vi "2ndStrikerNormal.vi"(5 "Stop":bool, 6 "atacando ao contrário?":bool=TRUE, 7 "AI Parameters":T1={"GotoKick"={"Dist do cone a frente"=150.0, "attacker farback"=1500.0, "Perto"=300.0, "min dist to kick"=150.0, "kick eps"=0.0, "Time to transition"=0.05}, "Attacker"={"CC chute"=0.09, "CC passe"=0.045, "Kick Force"=100.0, "ball-robot Kick"=200.0, "ball-robot Pass"=0.3, "drible\nAttk"=FALSE}, "Defender"={"D max"=1700.0, "Vel p/ robô av"=1000.0, "Kick Force"=100.0, "D atk-def"=0.0, "D farback"=0.0, "drible\ndef"=FALSE, "drible\ngoalie"=FALSE}, "Timeout"={"Field/v in x"=6.0, "Dist Robots"=300, "Dist up in y"=300}, "Pose Striker"={"dist"=200.0, "Numeric"=-4.0, "dist 2"=200.0, "drible\nstriker"=FALSE}, "Dist Stop"=300.0, "D ball out"=200, "D central gap "=150.0, "T pass"=0.0, "Force ++"=0.0, "range kick"=0.0, "Chute alto"=TRUE, "Marcador novo"=TRUE, "drible"=FALSE, "D drible"=300.0} {"D drible" format="%#_13g"; "D central gap" format="%#_13g"; "Dist Stop" format="%#_13g"; "Pose Striker"."Numeric" format="%#_13g"; "Defender"."Kick Force" format="%#_13g"; "Defender"."Vel p/ robô av" format="%#_13g"; "Attacker"."ball-robot Kick" format="%#_13g"; "Attacker"."Kick Force" format="%#_13g"; "Attacker"."CC passe" format="%#_13g"; "Attacker"."CC chute" format="%#_13g"; "GotoKick"."kick eps" format="%#_13g"; "GotoKick"."min dist to kick" format="%#_13g"; "GotoKick"."Perto" format="%#_13g"; "GotoKick"."attacker farback" format="%#_13g"; "GotoKick"."Dist do cone a frente" format="%#_13g"}, 8 "IA Input":T9={"our_robots"=[], "enemy_robots"=[], "balls"=[], "geometry"={"line_width"=0, "field_length"=0, "field_width"=0, "boundary_width"=0, "referee_width"=0, "goal_width"=0, "goal_depth"=0, "goal_wall_width"=0, "center_circle_radius"=0, "defense_radius"=0, "defense_stretch"=0, "free_kick_from_defense_dist"=0, "penalty_spot_from_field_line_dist"=0, "penalty_line_from_spot_dist"=0}, "IA Judge"={"stage"="", "command"="", "our_goalie_id"=0.0, "enemy_goalie_id"=0.0, "command enum"=enum."Halt", "Time"=enum."Azul"}, "Received Timestamp"=timestamp(0 s since 1904-01-01), "Events"={"Touch"=FALSE, "Ball out"=FALSE, "id touch"=0.0, "Ball out of \nVision"=FALSE, "Ball inside \nGoalie area"=FALSE, "Robot not responding"=FALSE, "Robots responding status"=[1.0, 1.0, 1.0, 1.0, 1.0, 1.0], "Enemy Ball \nPossession"=FALSE, "Pass State"=FALSE, "id end of pass"=0.0, "Kick"=FALSE, "Id ini Possession"=0.0, "Ball Possesion"=FALSE, "Id Possesion"=0.0, "Direct Kick"=FALSE, "2nd Strk Ativo"=FALSE}}, 9 "balls":T7[](array[typedef])=[{"x"=-2165.869384765625, "y"=510.4085693359375, "timestamp"=timestamp(2082758857.4639893 s since 1904-01-01), "Vel_x"=0.0, "Vel_y"=0.0, "Pos Bola Est"=[]}], 10 "Field Size in":T8={"line_width"=10, "field_length"=6000, "field_width"=4000, "boundary_width"=250, "referee_width"=425, "goal_width"=700, "goal_depth"=180, "goal_wall_width"=20, "center_circle_radius"=500, "defense_radius"=500, "defense_stretch"=350, "free_kick_from_defense_dist"=700, "penalty_spot_from_field_line_dist"=450, "penalty_line_from_spot_dist"=350}, 11 "Robot in":T2={"id"=5, "function"=enum."Attacker", "x"=-1842.5054931640625, "y"=520.60986328125, "orientation"=-2.7555055618286133, "v_tangent"=0.0, "v_normal"=0.0, "v_ang"=0.0, "kick_x"=0.0, "kick_z"=0.0, "dribble"=FALSE, "Timestamp"=timestamp(2082758857.4639893 s since 1904-01-01), "estimatives"={"est_v_tangent"=0.0, "est_v_normal"=0.0, "est_vx"=0.0, "est_vy"=0.0, "Pos Robot Est"=[]}, "dest_x_kick"=0.0, "dest_y_kick"=0.0, "Gap Coord"=[], "States"=enum."GoToTangent", "Path "=[], "Path  Smooth"=[], "Dest"=[]}) -> (2 "Robot out":T2={"id"=5, "function"=enum."Attacker", "x"=-1842.5054931640625, "y"=520.60986328125, "orientation"=-2.7555055618286133, "v_tangent"=-0.08361641967936218, "v_normal"=-0.20513016702014014, "v_ang"=0.24456003022714357, "kick_x"=0.0, "kick_z"=0.0, "dribble"=FALSE, "Timestamp"=timestamp(2082758857.4639893 s since 1904-01-01), "estimatives"={"est_v_tangent"=0.0, "est_v_normal"=0.0, "est_vx"=0.0, "est_vy"=0.0, "Pos Robot Est"=[]}, "dest_x_kick"=0.0, "dest_y_kick"=0.0, "Gap Coord"=[], "States"=enum."GoToTangent", "Path "=[], "Path  Smooth"=[], "Dest"=[]})   [LabVIEW 2017]
uses:
  Core/AI Robot.ctl
  Functions Enum.ctl
  AttackerStates.ctl
  Path Planning/RRT/PathDests.ctl
  Path Planning/RRT/PathDest.ctl
  Core/AI Input.ctl
  Core/AI Ball.ctl
  Core/Field Size.ctl
  Core/AI Judge.ctl
  Command Enum.ctl
  Util/Events/Events.ctl
  AI Parameters.ctl
panel:
  in  "Wait pass perpendicular?":bool=TRUE
  in  "Marcador sempre":bool
  out "size(s)":i32
  in  "IDattacker":dbl
  in  "Yattacker":dbl
  in  "Xattacker":dbl
  out "States":T4
  out "sentido":dbl
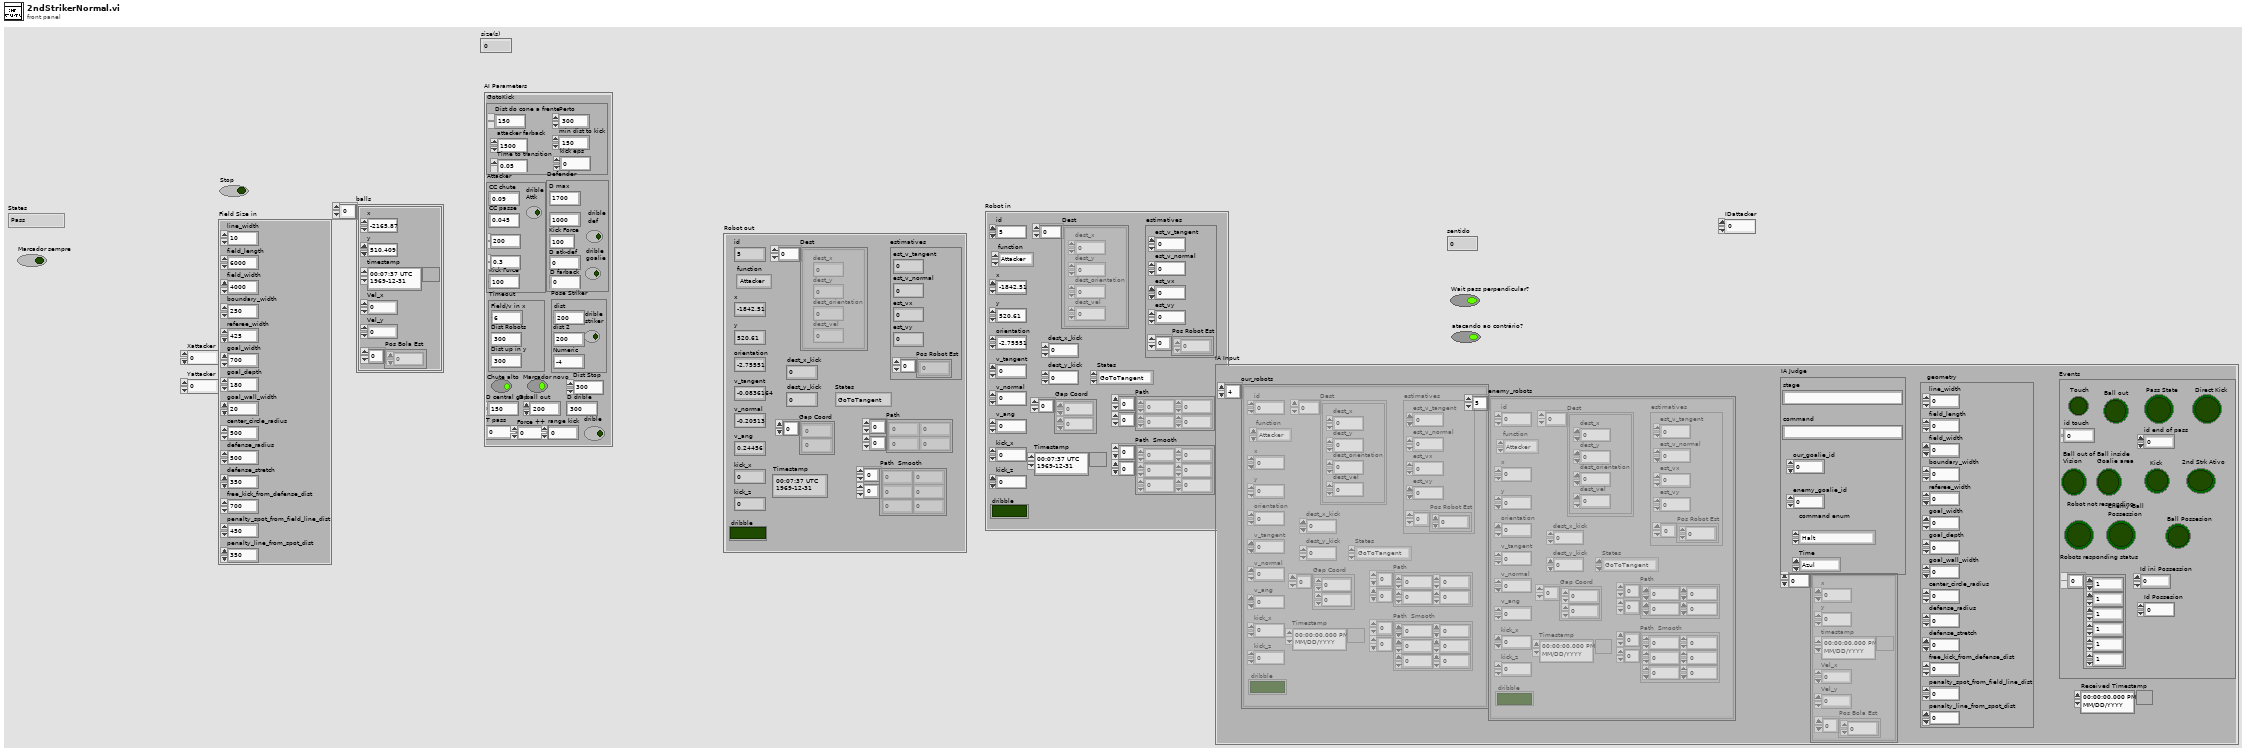
[diagram p1: front panel]
types:
  T1 = typedef "AI Parameters.ctl" = cluster{"GotoKick":cluster{"Dist do cone a frente":dbl, "attacker farback":dbl, "Perto":dbl, "min dist to kick":dbl, "kick eps":dbl, "Time to transition":dbl}, "Attacker":cluster{"CC chute":dbl, "CC passe":dbl, "Kick Force":dbl, "ball-robot Kick":dbl, "ball-robot Pass":dbl, "drible\nAttk":bool}, "Defender":cluster{"D max":dbl, "Vel p/ robô av":dbl, "Kick Force":dbl, "D atk-def":dbl, "D farback":dbl, "drible\ndef":bool, "drible\ngoalie":bool}, "Timeout":cluster{"Field/v in x":dbl, "Dist Robots":u32, "Dist up in y":u32}, "Pose Striker":cluster{"dist":dbl, "Numeric":dbl, "dist 2":dbl, "drible\nstriker":bool}, "Dist Stop":dbl, "D ball out":i32, "D central gap ":dbl, "T pass":dbl, "Force ++":dbl, "range kick":dbl, "Chute alto":bool, "Marcador novo":bool, "drible":bool, "D drible":dbl}
  T2 = typedef "AI Robot.ctl" = cluster{"id":u32, "function":T3, "x":dbl, "y":dbl, "orientation":dbl, "v_tangent":dbl, "v_normal":dbl, "v_ang":dbl, "kick_x":dbl, "kick_z":dbl, "dribble":bool, "Timestamp":timestamp, "estimatives":cluster{"est_v_tangent":dbl, "est_v_normal":dbl, "est_vx":dbl, "est_vy":dbl, "Pos Robot Est":dbl[]}, "dest_x_kick":dbl, "dest_y_kick":dbl, "Gap Coord":dbl[], "States":T4, "Path ":dbl[][], "Path  Smooth":dbl[][], "Dest":T5}
  T3 = typedef "Functions Enum.ctl" = enum16{"2nd Striker", "Attacker", "Goalie", "Defender", "Striker", "Goto 0", "Dummy", "Kicker", "ZigZag 0", "ZigZag 1", "ZigZag 2", "ZigZag 3", "ZigZag 4", "ZigZag 5", "ZigZag 6", "ZigZag 7", "ZigZag 8", ""}
  T4 = typedef "AttackerStates.ctl" = enum16{"Pass", "GoToTangent", "BallGetting", "GoToKick", ""}
  T5 = typedef "PathDests.ctl" = T6[]
  T6 = typedef "PathDest.ctl" = cluster{"dest_x":dbl, "dest_y":dbl, "dest_orientation":dbl, "dest_vel":dbl}
  T7 = typedef "AI Ball.ctl" = cluster{"x":dbl, "y":dbl, "timestamp":timestamp, "Vel_x":dbl, "Vel_y":dbl, "Pos Bola Est":dbl[]}
  T8 = typedef "Field Size.ctl" = cluster{"line_width":u32, "field_length":u32, "field_width":u32, "boundary_width":u32, "referee_width":u32, "goal_width":u32, "goal_depth":u32, "goal_wall_width":u32, "center_circle_radius":u32, "defense_radius":u32, "defense_stretch":u32, "free_kick_from_defense_dist":u32, "penalty_spot_from_field_line_dist":u32, "penalty_line_from_spot_dist":u32}
  T9 = typedef "AI Input.ctl" = cluster{"our_robots":T2[], "enemy_robots":T2[], "balls":T7[], "geometry":T8, "IA Judge":T10, "Received Timestamp":timestamp, "Events":T12}
  T10 = typedef "AI Judge.ctl" = cluster{"stage":string, "command":string, "our_goalie_id":dbl, "enemy_goalie_id":dbl, "command enum":T11, "Time":enum16{"Azul", "Amarelo"}}
  T11 = typedef "Command Enum.ctl" = enum16{"Halt", "Stop", "Force Start", "PKA Normal Start", "Prepare Kickoff Ally", "PKE Normal Start", "Prepare Kickoff Enemy", "Prepare Penalty Ally", "PPA Normal Start", "Prepare Penalty Enemy", "PPE Normal Start", "Direct Free Enemy", "Direct Free Ally", "Indirect Free Enemy", "Indirect Free Ally", "Timeout Enemy", "Timeout Ally", "Goal Enemy", "Goal Ally", "Ball Placement Enemy", "Ball Placement Ally", "Normal Half Time", "Extra Time Break", "Extra Half Time", "None", "Post Game"}
  T12 = typedef "Events.ctl" = cluster{"Touch":bool, "Ball out":bool, "id touch":dbl, "Ball out of \nVision":bool, "Ball inside \nGoalie area":bool, "Robot not responding":bool, "Robots responding status":dbl[], "Enemy Ball \nPossession":bool, "Pass State":bool, "id end of pass":dbl, "Kick":bool, "Id ini Possession":dbl, "Ball Possesion":bool, "Id Possesion":dbl, "Direct Kick":bool, "2nd Strk Ativo":bool}
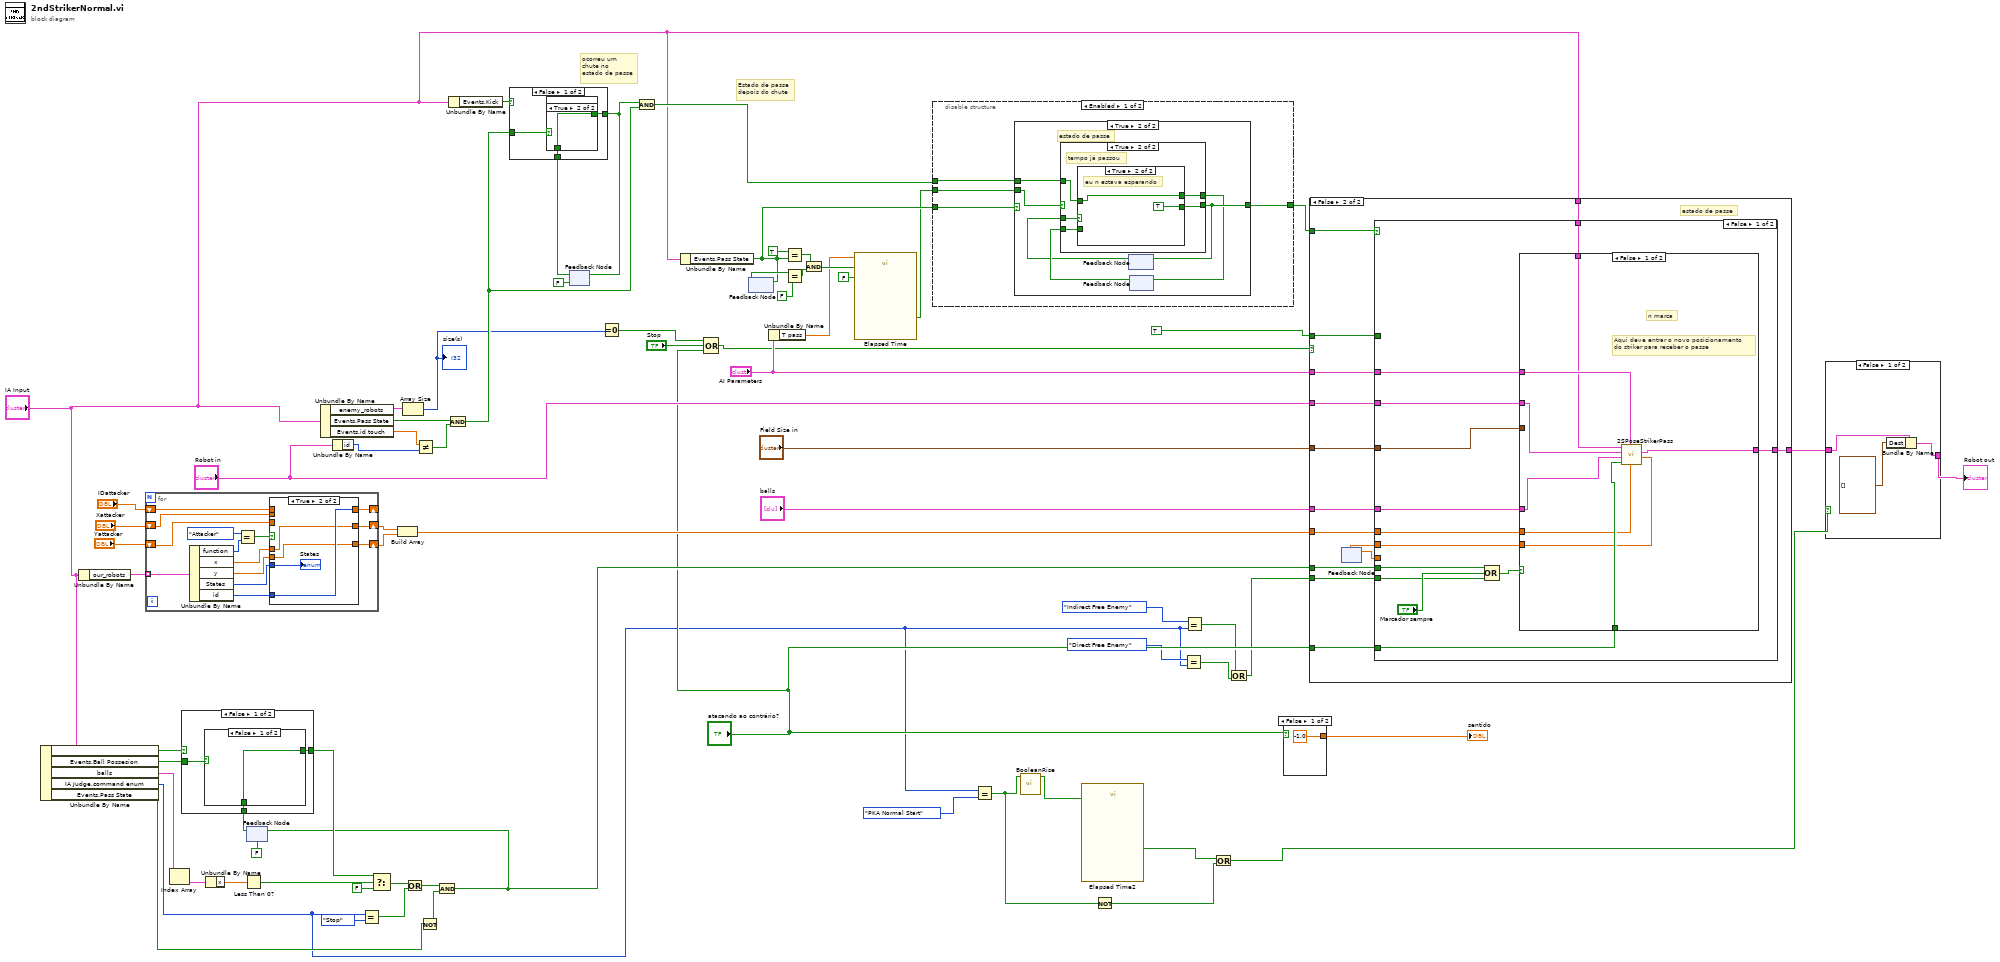
[diagram p0: block diagram]
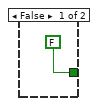
[diagram p3: hidden frame]
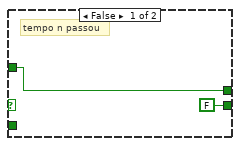
[diagram p4: hidden frame]
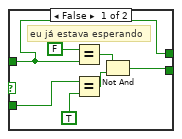
[diagram p5: hidden frame]
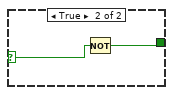
[diagram p7: hidden frame]
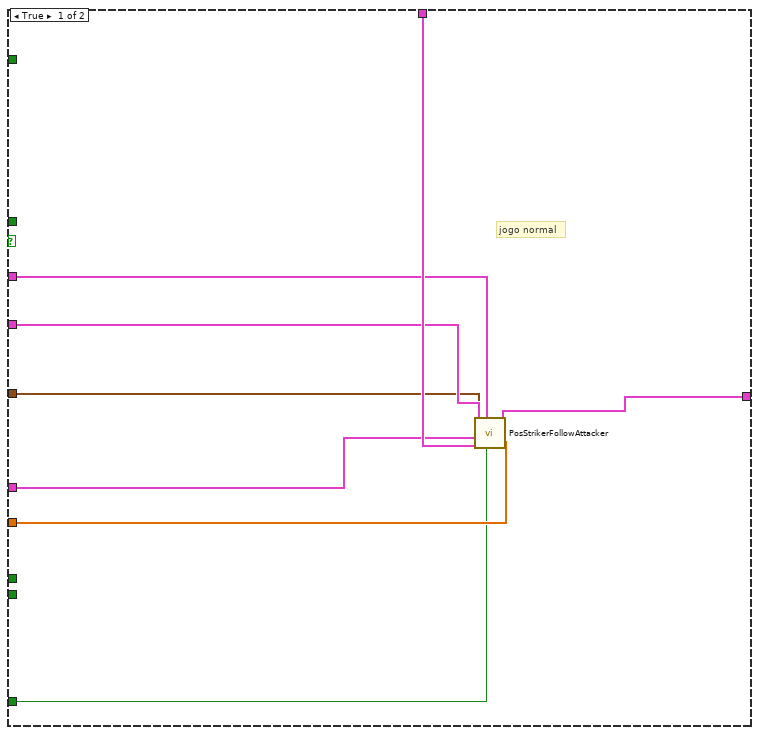
[diagram p9: hidden frame]
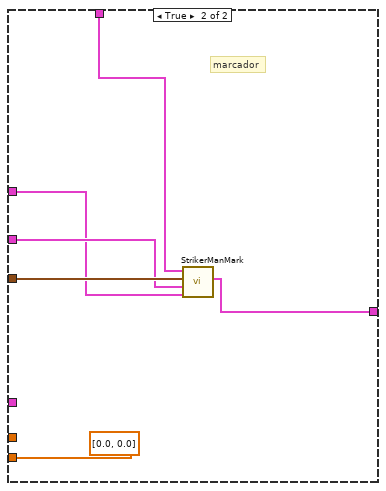
[diagram p10: hidden frame]
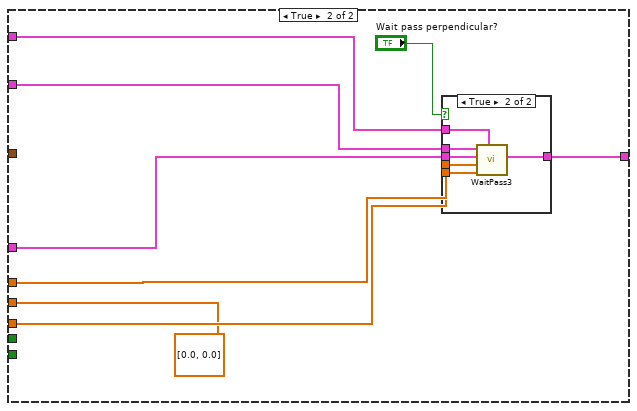
[diagram p11: hidden frame]
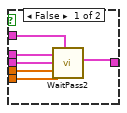
[diagram p12: hidden frame]
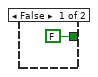
[diagram p14: hidden frame]
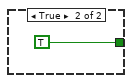
[diagram p15: hidden frame]
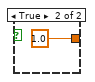
[diagram p16: hidden frame]
diagram:
  # "ocorreu um \nchute no\nestado de passe"
  # "Estado de passe\ndepois do chute"
  n1 = Unbundle By Name("IA Input") -> ("Events.Enemy Ball \nPossession"=w50:bool, "Events.Ball Possesion"=w49:bool, "balls"=w47:T7[], "IA Judge.command enum"=w9:T11, "Events.Pass State"=w37:bool)
  n2 = Unbundle By Name("IA Input") -> ("our_robots"=w66:T2[])
  n3 = for {
    tunnel: w66 -> [w81] mode=indexing
    shift-right: [w77] -> w62
    shift-left: "Xattacker" -> [w75]
    shift-right: [w76] -> w61
    shift-left: "Yattacker" -> [w74]
    shift-right: [w78] -> _
    shift-left: "IDattacker" -> [w73]
    n4 = Unbundle By Name(w81) -> ("function"=w86:T3, "x"=w83:dbl, "y"=w82:dbl, "States"=w80:T4, "id"=w79:u32)
    n5 = Equal?(x=Functions_Enum."Attacker", y=w86) -> (x = y?=w84:bool)
    n6 = case shown="True" w84 {
      tunnel: w83 -> [_ w91]
      tunnel: w82 -> [_ w90]
      tunnel: w80 -> [_ w93]
      tunnel: w79 -> [_ w92]
      tunnel: [w87 w92] -> w78
      tunnel: [w89 w91] -> w77
      tunnel: [w88 w90] -> w76
      tunnel: w75 -> [w89 _]
      tunnel: w74 -> [w88 _]
      tunnel: w73 -> [w87 _]
      frame False {
      }
      frame True {
        "States" <- w93
      }
    }
  }
  n7 = Index Array(array=w47) -> (element=w46:T7)  [unwired: 1 in]
  n8 = Unbundle By Name(w46) -> ("x"=w45:dbl)
  n9 = Less Than 0?(x=w45) -> (x < 0?=w44:bool)
  n10 = feedback #1(FALSE) -> (w48:bool)
  n11 = case shown="False" w50 {
    selector: w50 -> [_ w100]
    tunnel: [w95 w100] -> w43
    tunnel: w49 -> [w96 _]
    tunnel: w48 -> [w94 _]
    frame False {
      n12 = case shown="False" w96 {
        selector: w96 -> [_ w98]
        tunnel: [w97 w99] -> w95
        tunnel: w94 -> [w97 _]
        frame False {
        }
        frame True {
          n13 = Not(x=w98) -> (.not. x?=w99:bool)
        }
      }
    }
    frame True {
    }
  }
  n14 = Unbundle By Name("IA Input") -> ("enemy_robots"=w22:T2[], "Events.Pass State"=w67:bool, "Events.id touch"=w56:dbl)
  n15 = Unbundle By Name("Robot in") -> ("id"=w55:u32)
  n16 = Equal?(x=w9, y=Command_Enum."Stop") -> (x = y?=w40:bool)
  n17 = Select(t=w43, s=w44, f=FALSE) -> (s? t:f=w41:bool)
  n18 = Build Array(w62, w61) -> (w60:dbl[])
  n19 = Array Size(array=w22) -> (size(s)=w20:i32)
  "size(s)" <- w20
  n20 = Or(x=w41, y=w40) -> (x .or. y?=w38:bool)
  n21 = Not Equal?(x=w56, y=w55) -> (x != y?=w57:bool)
  n22 = Not(x=w37) -> (.not. x?=w36:bool)
  n23 = And(x=w38, y=w36) -> (x .and. y?=w35:bool)
  n24 = feedback-in #1(w35) -> ()
  n25 = Unbundle By Name("IA Input") -> ("Events.Kick"=w71:bool)
  n26 = Compound Arithmetic op=AND(w67, w57) -> (w58:bool)
  n27 = feedback #2(FALSE) -> (w69:bool)
  n28 = case shown="False" w71 {
    tunnel: [w102 TRUE] -> w70
    tunnel: w69 -> [w101 _]
    tunnel: w58 -> [w103 _]
    frame False {
      n29 = case shown="True" w103 {
        tunnel: [FALSE w105] -> w102
        tunnel: w101 -> [_ w105]
        frame False {
        }
        frame True {
        }
      }
    }
    frame True {
    }
  }
  n30 = feedback-in #2(w70) -> ()
  n31 = Equal To 0?(x=w20) -> (x = 0?=w21:bool)
  n32 = And(x=w70, y=w58) -> (x .and. y?=w26:bool)
  n33 = Unbundle By Name("IA Input") -> ("Events.Pass State"=w24:bool)
  n34 = Compound Arithmetic op=OR(w21, "Stop", "atacando ao contrário?") -> (w17:bool)
  n35 = feedback #3() -> (w34:bool)  [unwired: 1 in]
  n36 = feedback-in #3(w24) -> ()
  n37 = Unbundle By Name("AI Parameters") -> ("T pass"=w18:dbl)
  n38 = Equal?(x=TRUE, y=w24) -> (x = y?=w30:bool)
  n39 = Equal?(x=w34, y=FALSE) -> (x = y?=w31:bool)
  n40 = And(x=w30, y=w31) -> (x .and. y?=w29:bool)
  n41 = call "Elapsed Time"("Time Target (s)"=w18, "Reset"=w29, "Auto Reset"=FALSE) -> ("Time has Elapsed"=w23:bool)  [unwired: 9 in, 7 out]
  n42 = disable-structure shown="Enabled" {
    disable-tunnel: w23 -> [w108 _]
    disable-tunnel: [w110 w134] -> w27
    disable-tunnel: w26 -> [w109 w134]
    disable-tunnel: w24 -> [w107 _]
    frame Enabled {
      n43 = case shown="True" w107 {
        tunnel: [FALSE w117] -> w110
        tunnel: w109 -> [_ w116]
        tunnel: w108 -> [_ w113]
        frame False {
        }
        frame True {
          # "estado de passe"
          n44 = feedback #4() -> (w112:bool)  [unwired: 1 in]
          n45 = feedback #5() -> (w114:bool)  [unwired: 1 in]
          n46 = case shown="True" w113 {
            tunnel: [FALSE w123] -> w117
            tunnel: w116 -> [w118 w122]
            tunnel: [w118 w120] -> w115
            tunnel: w114 -> [_ w121]
            tunnel: w112 -> [_ w124]
            frame False {
              # "tempo n passou"
            }
            frame True {
              # "tempo já passou"
              n47 = case shown="True" w124 {
                tunnel: [w126 TRUE] -> w123
                tunnel: w122 -> [w125 w132]
                tunnel: w121 -> [w127 _]
                tunnel: [w125 w132] -> w120
                frame False {
                  # "eu já estava esperando"
                  n48 = Equal?(x=FALSE, y=w125) -> (x = y?=w128:bool)
                  n49 = Equal?(x=w127, y=TRUE) -> (x = y?=w129:bool)
                  n50 = Not And(1:w129, 2:w128) -> (0:w126:bool)
                }
                frame True {
                  # "eu n estava esperando"
                }
              }
            }
          }
          n51 = feedback-in #4(w117) -> ()
          n52 = feedback-in #5(w115) -> ()
        }
      }
    }
    frame Disabled {
    }
  }
  n53 = Equal?(x=w9, y=Command_Enum."PKA Normal Start") -> (x = y?=w4:bool)
  n54 = call "BooleanRise.vi"("Test Mode On"=w4) -> ("Boolean"=w7:bool)  [unwired: 10 in]
  n55 = call "Elapsed Time2"("Reset"=w7) -> ("Time has Elapsed"=w2:bool)  [unwired: 11 in, 7 out]
  n56 = Not(x=w4) -> (.not. x?=w3:bool)
  n57 = Equal?(x=Command_Enum."Direct Free Enemy", y=w9) -> (x = y?=w12:bool)
  n58 = Equal?(x=Command_Enum."Indirect Free Enemy", y=w9) -> (x = y?=w11:bool)
  n59 = Or(x=w2, y=w3) -> (x .or. y?=w1:bool)
  n60 = Compound Arithmetic op=OR(w11, w12) -> (w10:bool)
  n61 = case shown="False" "atacando ao contrário?" {
    tunnel: [-1.0 1.0] -> w72
    frame False {
    }
    frame True {
    }
  }
  "sentido" <- w72
  n62 = case shown="False" w17 {
    tunnel: w27 -> [_ w150]
    tunnel: TRUE -> [_ w151]
    tunnel: "Robot in" -> [w143 w158]
    tunnel: w60 -> [w140 w157]
    tunnel: "atacando ao contrário?" -> [w139 w156]
    tunnel: "Field Size in" -> [w142 w155]
    tunnel: "balls" -> [w141 w154]
    tunnel: "IA Input" -> [w144 w153]
    tunnel: [w138 w152] -> w5
    tunnel: "AI Parameters" -> [w137 w149]
    tunnel: w35 -> [_ w148]
    tunnel: w10 -> [_ w145]
    frame True {
      # "jogo normal"
      n63 = call "PosStrikerFollowAttacker.vi"("Pos Attacker"=w140, "atacando ao contrário?"=w139, "AI Parameters"=w137, "IA Input"=w144, "balls"=w141, "Field Size in"=w142, "Robot in"=w143) -> ("Robot out"=w138:T2)  [unwired: 4 in]
    }
    frame False {
      # "estado de passe"
      n64 = feedback #6() -> (w146:dbl[])  [unwired: 1 in]
      n65 = case shown="False" w150 {
        tunnel: w151 -> [_ _]
        tunnel: w158 -> [w170 w193]
        tunnel: w157 -> [w165 w192]
        tunnel: [w167 w191] -> w152
        tunnel: w156 -> [w171 _]
        tunnel: w155 -> [w164 _]
        tunnel: w154 -> [w169 w190]
        tunnel: w153 -> [w168 _]
        tunnel: w149 -> [w166 w186]
        tunnel: w148 -> [w163 _]
        tunnel: [w160 dbl[] [0.0, 0.0] ("FinalPosition")] -> w147
        tunnel: w146 -> [_ w189]
        tunnel: w145 -> [w159 _]
        frame False {
          n66 = Compound Arithmetic op=OR(w163, "Marcador sempre", w159) -> (w162:bool)
          n67 = case shown="False" w162 {
            tunnel: w171 -> [w175 _]
            tunnel: w170 -> [w177 w184]
            tunnel: w169 -> [w174 _]
            tunnel: w168 -> [w176 w182]
            tunnel: [w179 w183] -> w167
            tunnel: w166 -> [w178 w181]
            tunnel: w165 -> [w173 _]
            tunnel: w164 -> [_ w185]
            tunnel: [w172 dbl[] [0.0, 0.0] ("FinalPosition")] -> w160
            frame False {
              # "n marca"
              # "Aqui deve entrar o novo posicionamento\ndo striker para receber o passe"
              n68 = call "2SPoseStrikerPass.vi"("Array"=w173, "AI Parameters"=w178, "atacando ao contrário?"=w175, "balls"=w174, "Robot in"=w177, "IA Input"=w176) -> ("FinalPosition"=w172:dbl[], "Robot out"=w179:T2)  [unwired: 4 in]
            }
            frame True {
              # "marcador"
              n69 = call "StrikerManMark.vi"("AI Parameters"=w181, "Robot in"=w184, "Field Size in"=w185, "IA Input"=w182) -> ("Robot out"=w183:T2)  [unwired: 6 in, 1 out]
            }
          }
        }
        frame True {
          n70 = case shown="True" "Wait pass perpendicular?" {
            tunnel: w193 -> [w198 w205]
            tunnel: w192 -> [w196 w204]
            tunnel: [w199 w203] -> w191
            tunnel: w190 -> [w197 w202]
            tunnel: w189 -> [w195 w201]
            tunnel: w186 -> [w194 w200]
            frame False {
              n71 = call "WaitPass2.vi"("AI Parameters"=w194, "Best Y Inverso"=w195, "Target"=w196, "balls"=w197, "Robot in"=w198) -> ("Robot out"=w199:T2)  [unwired: 6 in]
            }
            frame True {
              n72 = call "WaitPass3.vi"("AI Parameters"=w200, "Best Y Inverso"=w201, "Target"=w204, "balls"=w202, "Robot in"=w205) -> ("Robot out"=w203:T2)  [unwired: 6 in]
            }
          }
        }
      }
      n73 = feedback-in #6(w147) -> ()
    }
  }
  n74 = case shown="False" w1 {
    tunnel: [w207 w209] -> w6
    tunnel: w5 -> [w208 w209]
    frame False {
      n75 = Bundle By Name(cluster=w208, "Dest"=T5 []) -> (w207:T2)
    }
    frame True {
    }
  }
  "Robot out" <- w6
